vi "Post Command.vi"(6 "timeout in ms (-1)":i32, 7 "Priority?":bool, 8 "error in (no error)":errorcluster, 9 "Data":variant, 10 "Command":string, 11 "queue in":refnum<queue>) -> (0 "error out":errorcluster, 3 "queue out":refnum<queue>, 4 "timed out?":bool)   [LabVIEW 2012, in "Cmd Queue.lvlib"]
uses:
  Cmd Queue.lvlib
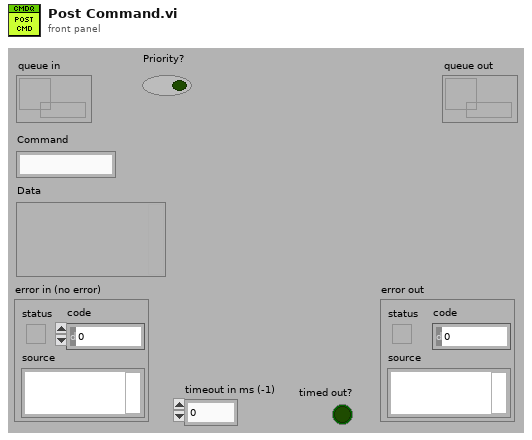
[diagram p1: front panel]
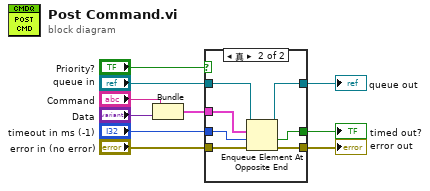
[diagram p0: block diagram]
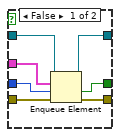
[diagram p2: hidden frame]
diagram:
  n1 = Bundle("Command"="Command", "Data"="Data") -> (w4:cluster{"Command":string, "Data":variant})  [unwired: 1 in]
  n2 = case shown="真" "Priority?" {
    tunnel: "queue in" -> [w17 w24]
    tunnel: "timeout in ms (-1)" -> [w16 w23]
    tunnel: [w15 w22] -> w8
    tunnel: [w14 w21] -> w7
    tunnel: w4 -> [w13 w20]
    tunnel: "error in (no error)" -> [w12 w19]
    tunnel: [w11 w18] -> w2
    frame False {
      n3 = Enqueue Element(queue=w17, element=w13, timeout in ms (-1)=w16, error in (no error)=w12) -> (queue out=w15:refnum<queue>, timed out?=w11:bool, error out=w14:errorcluster)
    }
    frame True {
      n4 = Enqueue Element At Opposite End(queue=w24, element=w20, timeout in ms (-1)=w23, error in (no error)=w19) -> (queue out=w22:refnum<queue>, timed out?=w18:bool, error out=w21:errorcluster)
    }
  }
  "error out" <- w7
  "queue out" <- w8
  "timed out?" <- w2
